vi "Read Helper Stop Notifier.vi"(8 "error in (no error)":errorcluster, 11 "Mock Process In":refnum<class "Mock Process.lvclass">) -> (0 "error out":errorcluster, 2 "Helper Stopped Notifier":refnum<notifier>, 3 "Mock Process Out":refnum<class "Mock Process.lvclass">)   [LabVIEW 2020, in "Mock Process.lvclass"]
doc: "Framework method for getting the notifier used to stop the helper loop and provide handshake that the loop has stopped."
uses:
  Mock Process.lvclass
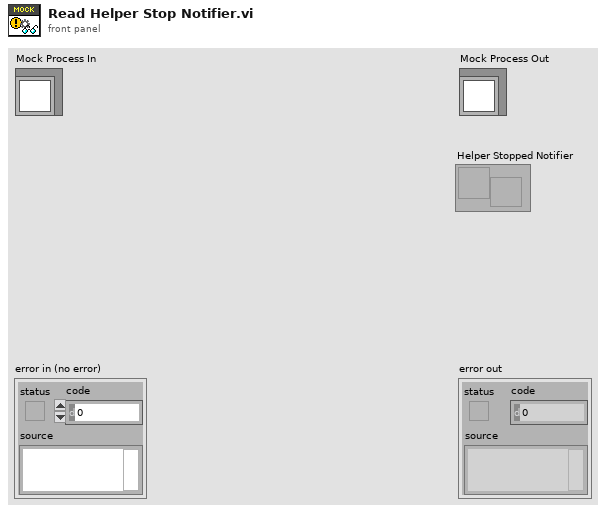
[diagram p1: front panel]
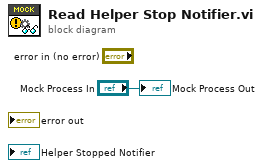
[diagram p0: block diagram]
diagram:
  "Mock Process Out" <- "Mock Process In"
